vi "p6100_write_setpoint.vi"(0 "VISA in":refnum<visa-resource-name>, 1 "Serial Parameters":T1, 2 "Setpoint":cluster{dbl, dbl}, 3 "error in":errorcluster) -> (5 "VISA out":refnum<visa-resource-name>, 6 "Temp":cluster{"Bottom":dbl, "Top":dbl}, 7 "error out":errorcluster)   [LabVIEW 2011]
uses:
  <vilib>/NI Modbus.llb/MB Serial Master Query Write Single Register (poly).vi
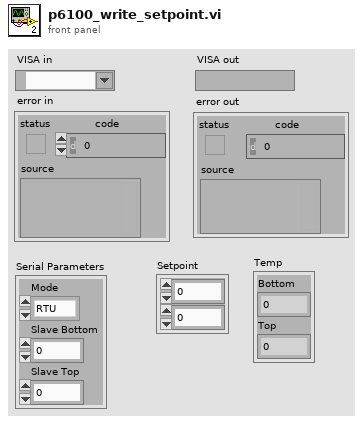
[diagram p1: front panel]
types:
  T1 = cluster{"Mode":enum16{"RTU", "ASCII"}, "Slave Bottom":u8, "Slave Top":u8}
  T2 = cluster{"Mode":enum16{"RTU", "ASCII"}, "Slave Bottom":u8}
  T3 = cluster{"Mode":enum16{"RTU", "ASCII"}, "Slave Top":u8}
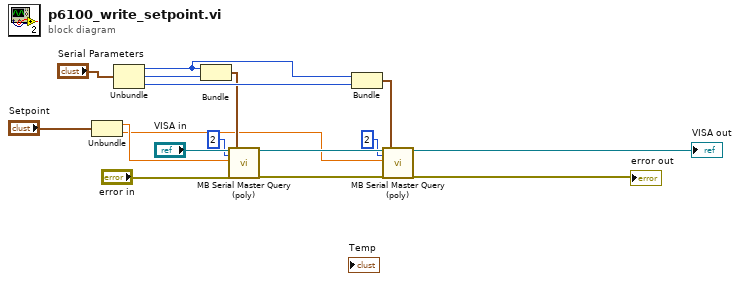
[diagram p0: block diagram]
diagram:
  n1 = Unbundle("Setpoint") -> (w3:dbl, w2:dbl)
  n2 = Unbundle("Serial Parameters") -> ("Mode"=w10:enum16{"RTU", "ASCII"}, "Slave Bottom"=w12:u8, "Slave Top"=w11:u8)
  n3 = Bundle("Mode"=w10, "Slave Bottom"=w12) -> (w9:T2)  [unwired: 1 in]
  n4 = call-poly <vilib>:"MB Serial Master Query (poly).vi"("VISA resource name"="VISA in", "Address"=u16 2, "Holding Register"=w3, "error in"="error in", "Serial Parameters"=w9) -> ("VISA resource name out"=w17:refnum<visa-resource-name>, "error out"=w16:errorcluster)  [unwired: 12 in, 1 out]
  n5 = Bundle("Mode"=w10, "Slave Top"=w11) -> (w8:T3)  [unwired: 1 in]
  n6 = call-poly <vilib>:"MB Serial Master Query (poly).vi"("VISA resource name"=w17, "Address"=u16 2, "Holding Register"=w2, "error in"=w16, "Serial Parameters"=w8) -> ("VISA resource name out"=→"VISA out":refnum<visa-resource-name>, "error out"=→"error out":errorcluster)  [unwired: 12 in, 1 out]
